vi "DoExperiment.vi"(8 "Error In":errorcluster, 9 "Camera Information 2":T3 {"VS Speed (us)" format="%.2f"}, 10 "Acquisition Parameters":T4={"Acquisition Mode"=enum."Single Scan", "Trigger Mode"=enum."Internal", "Frame \nTransfer"=FALSE, "Exposure Time (s)"=0.0, "Accumulation Cycle Time (s)"=0.0, "# Accumulations"=1, "# Kinetics"=1, "Kinetic Cycle Time (s)"=0.0, "Horizontal Bin Size"=1, "Vertical Bin Size"=1} {"Vertical Bin Size" min=1; "Horizontal Bin Size" min=1; "Kinetic Cycle Time (s)" format="%.2f"; "# Kinetics" min=1; "# Accumulations" min=1; "Accumulation Cycle Time (s)" format="%.2f"; "Exposure Time (s)" format="%.2e"}, 11 "output cluster":T2) -> (0 "error out":errorcluster, 1 "Background Image":i32[][](graph), 2 "Atom Image":i32[][](graph), 3 "output cluster 2":T2)   [LabVIEW 2013]
uses:
  6704/6704_static_voltages_control.ctl
  AndorCamera/camera_controls.ctl
  <userlib>/atmcd32d.llb/AcquisitionMode_mode typedef.ctl
  <userlib>/atmcd32d.llb/TriggerMode_mode typedef.ctl
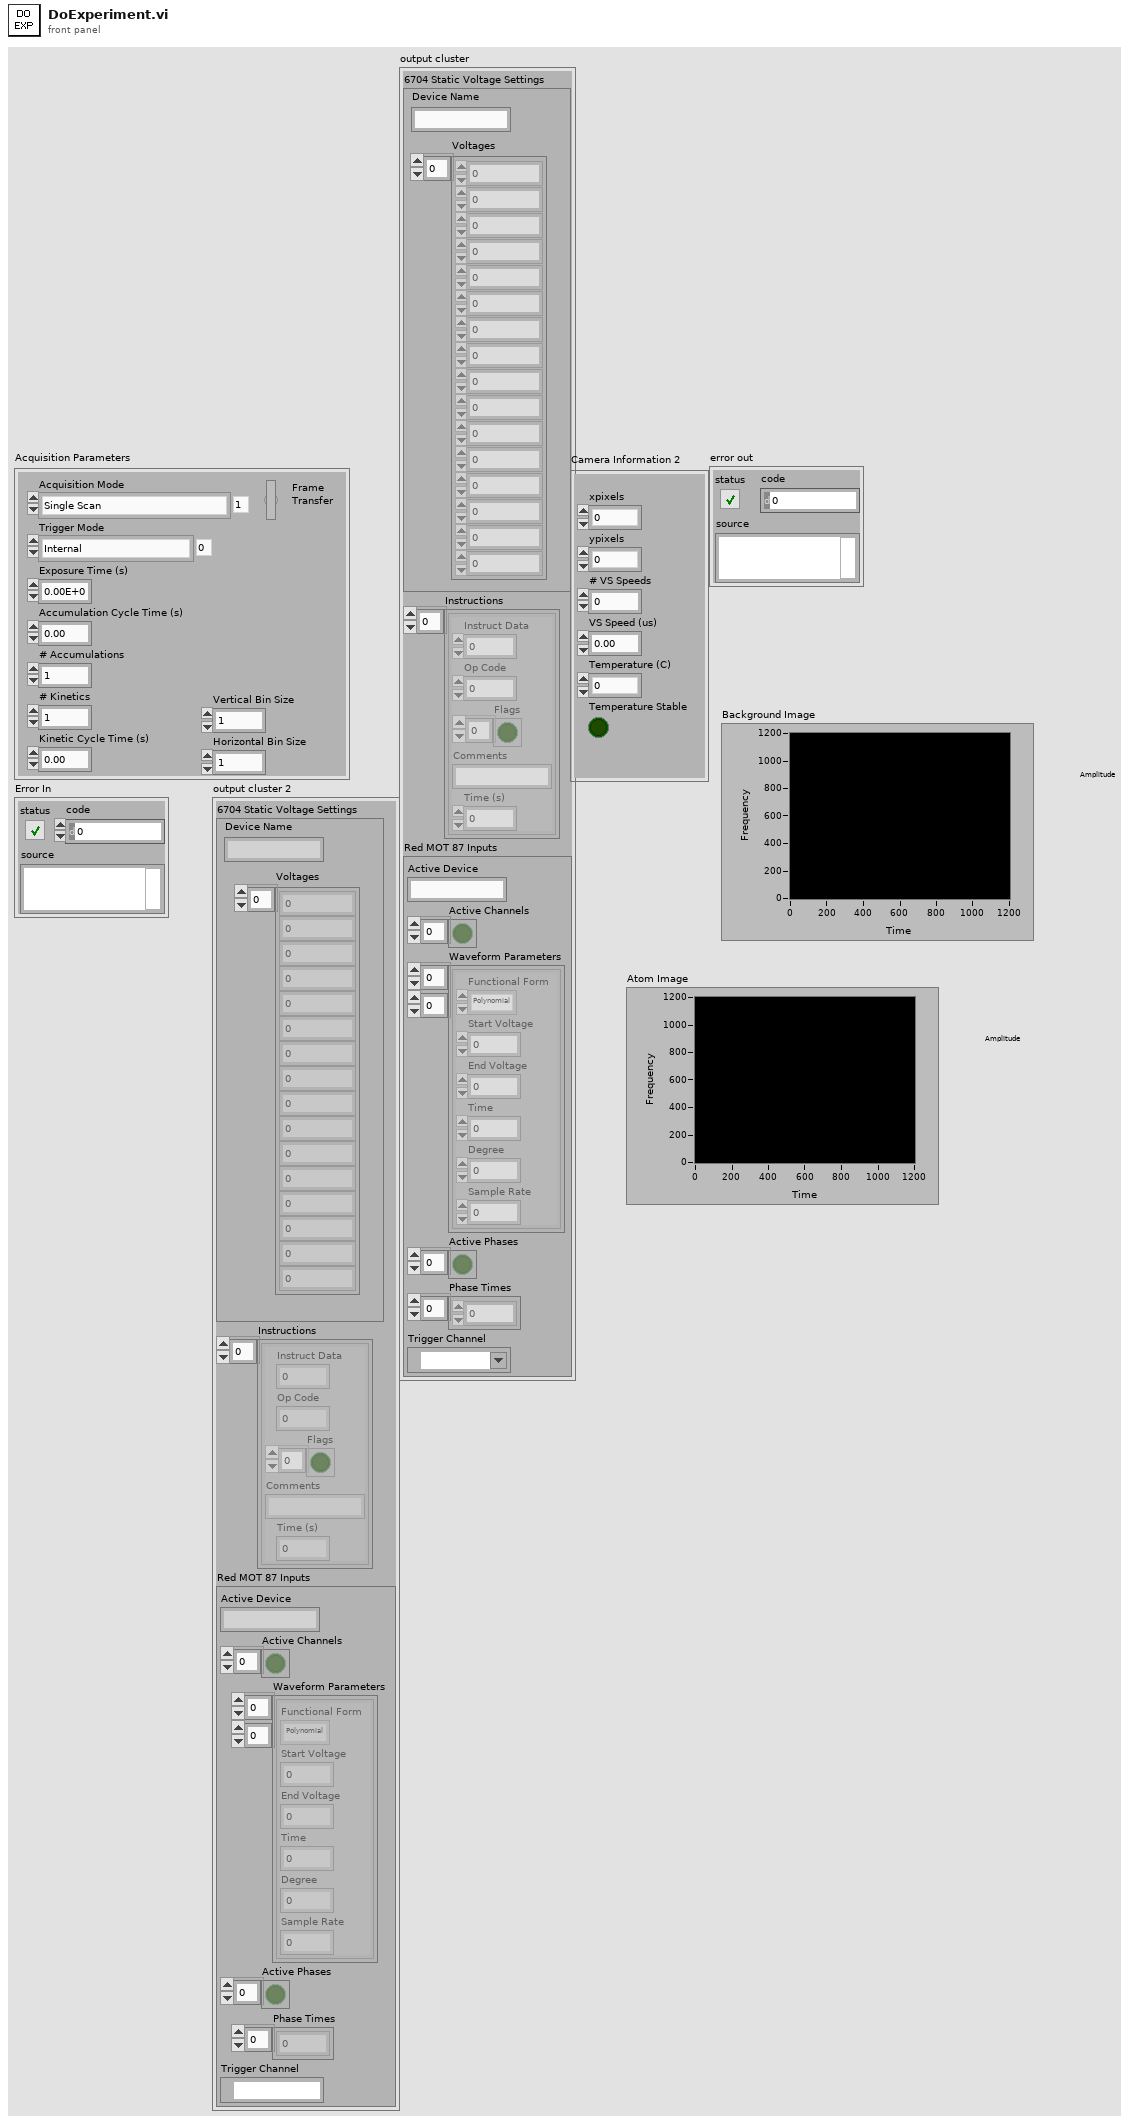
[diagram p1: front panel]
types:
  T1 = typedef "6704_static_voltages_control.ctl" = cluster{"Device Name":string, "Voltages":dbl[]}
  T2 = cluster{"6704 Static Voltage Settings":T1, "Instructions":cluster{"Instruct Data":i32, "Op Code":i32, "Flags":bool[], "Comments":string, "Time (s)":dbl}[], "Red MOT 87 Inputs":cluster{"Active Device":string, "Active Channels":bool[], "Waveform Parameters":cluster{"Functional Form":enum16{"Polynomial", "Exponential"}, "Start Voltage":dbl, "End Voltage":dbl, "Time":dbl, "Degree":i8, "Sample Rate":dbl}[][], "Active Phases":bool[], "Phase Times":dbl[], "Trigger Channel":tag}}
  T3 = cluster{"xpixels":i32, "ypixels":i32, "# VS Speeds":i32, "VS Speed (us)":sgl, "Temperature Stable":bool, "Temperature (C)":i32}
  T4 = typedef "camera_controls.ctl" = cluster{"Acquisition Mode":T5, "Trigger Mode":T6, "Frame \nTransfer":bool, "Exposure Time (s)":sgl, "Accumulation Cycle Time (s)":sgl, "# Accumulations":i32, "# Kinetics":i32, "Kinetic Cycle Time (s)":sgl, "Horizontal Bin Size":i32, "Vertical Bin Size":i32}
  T5 = typedef "AcquisitionMode_mode typedef.ctl" = enum16{"Reserved (0)", "Single Scan", "Accumulate", "Kinetics", "Fast Kinetics", "Run Till Abort", "Reserved (6)", "Reserved (7)", "Reserved (8)", "Time Delayed Integration"}
  T6 = typedef "TriggerMode_mode typedef.ctl" = enum16{"Internal", "External", "N/A (2)", "N/A (3)", "N/A (4)", "N/A (5)", "External Start", "External Exposure (Bulb)", "N/A (8)", "External FVB EM", "Software", "N/A (11)", "External Charge Shifting"}
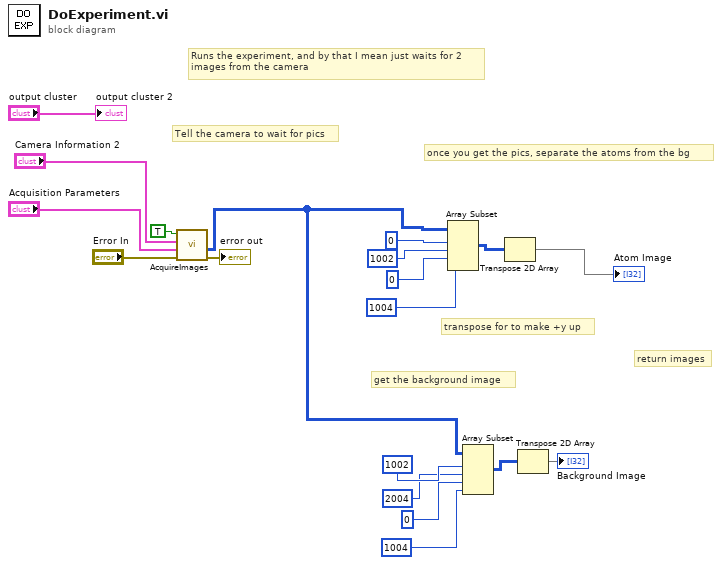
[diagram p0: block diagram]
diagram:
  # "return images"
  # "transpose for to make +y up"
  # "get the background image"
  # "once you get the pics, separate the atoms from the bg"
  # "Tell the camera to wait for pics"
  # "Runs the experiment, and by that I mean just waits for 2\nimages from the camera"
  n1 = call "AcquireImages.vi"("Error In"="Error In", "Acquisition Parameters"="Acquisition Parameters", "Camera Information 2"="Camera Information 2", "Pre Initialized?"=TRUE) -> ("error out"=→"error out":errorcluster, "Intensity Graph"=w2:i32[][])  [unwired: 6 in]
  n2 = Array Subset(array=w2, index (row)=0, length (row)=1002 ("length"), index (col)=0 ("index"), length (col)=1004 ("length")) -> (w4:i32[][])
  n3 = Array Subset(array=w2, index (row)=1002, length (row)=2004 ("length"), index (col)=0 ("index"), length (col)=1004 ("length")) -> (w5:i32[][])
  n4 = Transpose 2D Array(2D array=w4) -> (transposed array=→"Atom Image":i32[][])
  n5 = Transpose 2D Array(2D array=w5) -> (transposed array=→"Background Image":i32[][])
  "output cluster 2" <- "output cluster"
